vi "Set Cooler Power Status.vi"(8 "error in (no error)":errorcluster, 11 "CCDCamera in":refnum<class "CCDCamera.lvclass">) -> (0 "error out":errorcluster, 3 "CCDCamera out":refnum<class "CCDCamera.lvclass">)   [LabVIEW 2018, in "CCDCamera.lvclass"]
uses:
  CCDCamera.lvclass
  C:/Users/observer/Desktop/SPARC4_ACS/SPARC4_ACS/Simulated_CCD_Camera/Simulated_CCD_Camera.lvclass
  Simulated_CCD_Camera/Simulated_CCD_Camera.lvclass
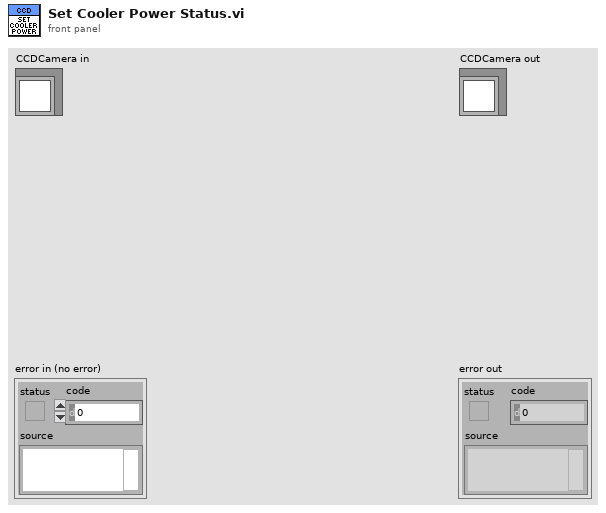
[diagram p1: front panel]
types:
  T1 = cluster{"COOLER_POWER_STATUS":u16, "TEMP":i32, "EXPTIME":sgl, "#FRAMES":u32, "#CUBES":u32, "COMMENT":string, "OBSTYPE":string, "OBJECT":string, "OBSERVER":string, "FILTER":string, "CTRLINTE":string}
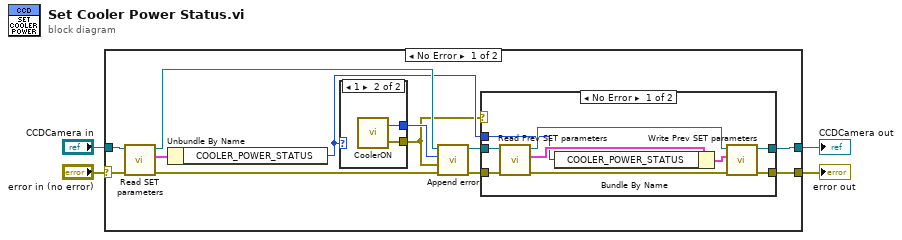
[diagram p0: block diagram]
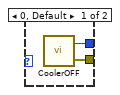
[diagram p3: hidden frame]
diagram:
  n1 = case shown="No Error" "error in (no error)" {
    selector: "error in (no error)" -> [w15 w32]
    tunnel: "CCDCamera in" -> [w16 w33]
    tunnel: [w7 w33] -> w2
    tunnel: [w8 w32] -> w1
    frame No Error {
      n2 = call-dynamic "Read SET parameters.vi"("error in (no error)"=w15, "Simulated_CCD_Camera in"=w16) -> ("error out"=w12:errorcluster, "New SET parameters"=w14:T1, "Simulated_CCD_Camera out"=w13:refnum<class "CCDCamera.lvclass">)  [unwired: 7 in]
      n3 = Unbundle By Name(w14) -> ("COOLER_POWER_STATUS"=w6:u16)
      n4 = case shown="1" w6 {
        tunnel: [w29 w31] -> w5
        tunnel: [w28 w30] -> w11
        frame 0, Default {
          n5 = call <userlib>:"CoolerOFF.vi"() -> ("error out"=w29:errorcluster, "DLL error code"=w28:u32)  [unwired: 2 in]
        }
        frame 1 {
          n6 = call <userlib>:"CoolerON.vi"() -> ("error out"=w31:errorcluster, "DLL error code"=w30:u32)  [unwired: 2 in]
        }
      }
      n7 = call "Append error.vi"("error in (no error)"=w12, "error"=w5, "code"=w11, "Simulated_CCD_Camera in"=w13) -> ("error out"=w9:errorcluster, "Simulated_CCD_Camera out"=w10:refnum<class "CCDCamera.lvclass">)  [unwired: 6 in]
      n8 = case shown="No Error" w5 {
        tunnel: [w25 w27] -> w7
        tunnel: [w24 w26] -> w8
        tunnel: w10 -> [w20 w27]
        tunnel: w9 -> [w21 w26]
        tunnel: w6 -> [w17 _]
        frame No Error {
          n9 = call-dynamic "Read Prev SET parameters.vi"("error in (no error)"=w21, "Simulated_CCD_Camera in"=w20) -> ("error out"=w22:errorcluster, "Old SET parameters"=w19:T1, "Simulated_CCD_Camera out"=w23:refnum<class "CCDCamera.lvclass">)  [unwired: 7 in]
          n10 = Bundle By Name(cluster=w19, "COOLER_POWER_STATUS"=w17) -> (w18:T1)
          n11 = call-dynamic "Write Prev SET parameters.vi"("error in (no error)"=w22, "Old SET parameters"=w18, "Simulated_CCD_Camera in"=w23) -> ("error out"=w24:errorcluster, "Simulated_CCD_Camera out"=w25:refnum<class "CCDCamera.lvclass">)  [unwired: 7 in]
        }
        frame Error {
        }
      }
    }
    frame Error {
    }
  }
  "error out" <- w1
  "CCDCamera out" <- w2
